vi "Actor Core.vi"(8 "error in":errorcluster caption="错误输入", 11 "Dialogue in":refnum<class "Dialogue.lvclass"> caption="操作者输入") -> (0 "error out":errorcluster caption="错误输出", 3 "Actor out":refnum<class "Actor.lvclass"> caption="操作者输出")   [LabVIEW 2014, in "Dialogue.lvlib" / "Dialogue.lvclass"]
doc: "(<B>文件名</B>：Actor Framework.lvlib:Actor.lvclass:Actor Core.vi)\n\n接收发送至操作者的消息，响应消息并处理可能导致操作者关闭的错误。\n\n子孙类重写该VI，使操作者完成特定的任务。使用调用父方法节点实现重写。"
uses:
  Dialogue.lvclass
  <vilib>/ActorFramework/Actor/Actor.lvclass
  <vilib>/ActorFramework/Actor/Actor.lvclass/Actor.ctl
  Dialogue.lvclass/Dialogue.ctl
  <vilib>/ActorFramework/Message Enqueuer/Message Enqueuer.lvclass/Message Enqueuer.ctl
  <vilib>/ActorFramework/Message Enqueuer/Enqueue.vi
  <vilib>/ActorFramework/Message Priority Queue/Priority Enqueue.vi
panel:
  out "格式化机器人指令":string[][](array[string])
  out "系统回应 4":string caption="标准输出"
  out "CM #":i32=-1
  out "显示窗口":string
  out "系统回应 3":string caption="标准输出"
  out "系统回应 2":string caption="标准输出"
  out "系统回应":string caption="标准输出"
  in  "重来":bool
  out "InstructionIn":string
  out "语音信号输出字符串":string
  in  "停止信号":bool
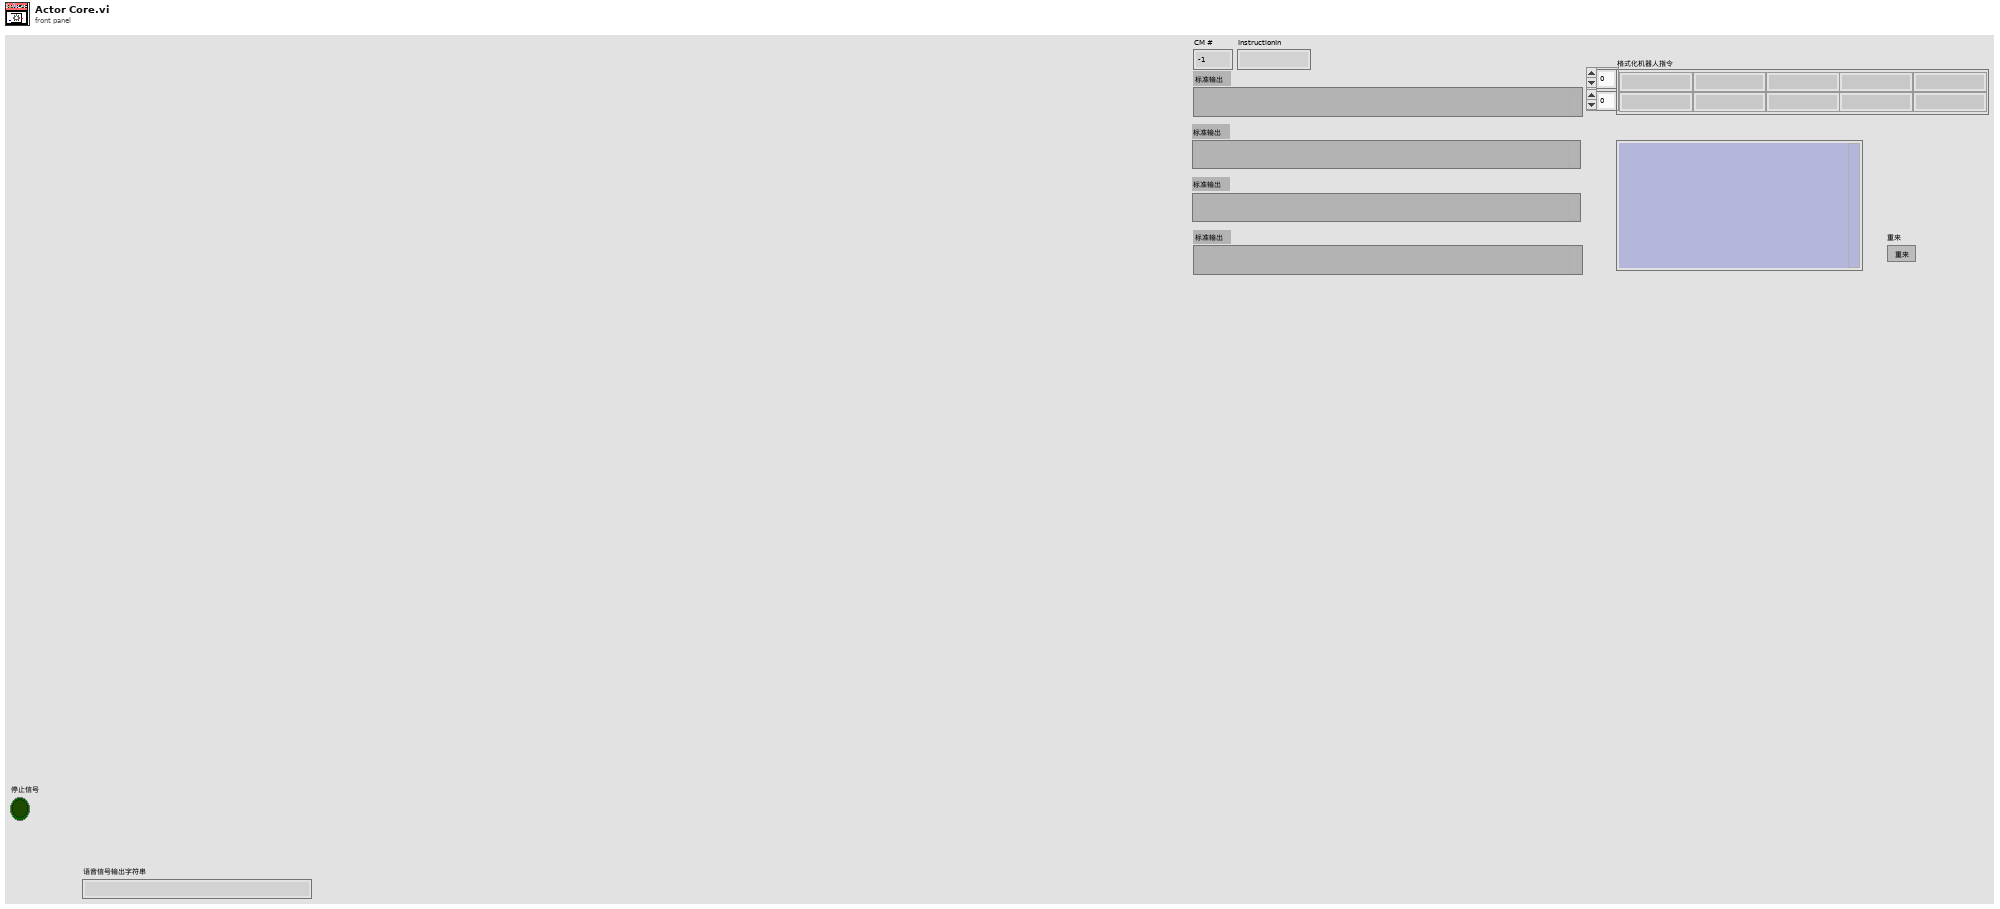
[diagram p1: front panel]
types:
  T1 = cluster{"输出数组":string[][], "CM #":i32, i32, string}
  T2 = cluster{"Stop":refnum<user-event>, "Text":refnum<user-event>, "Connected":refnum<user-event>}
  T3 = enum16{"open", "replace", "create", "open or create", "replace or create", "replace or create with confirmation"}
  T4 = cluster{"输出数组":string[][], "CM #":i32, "CM #":i32, string}
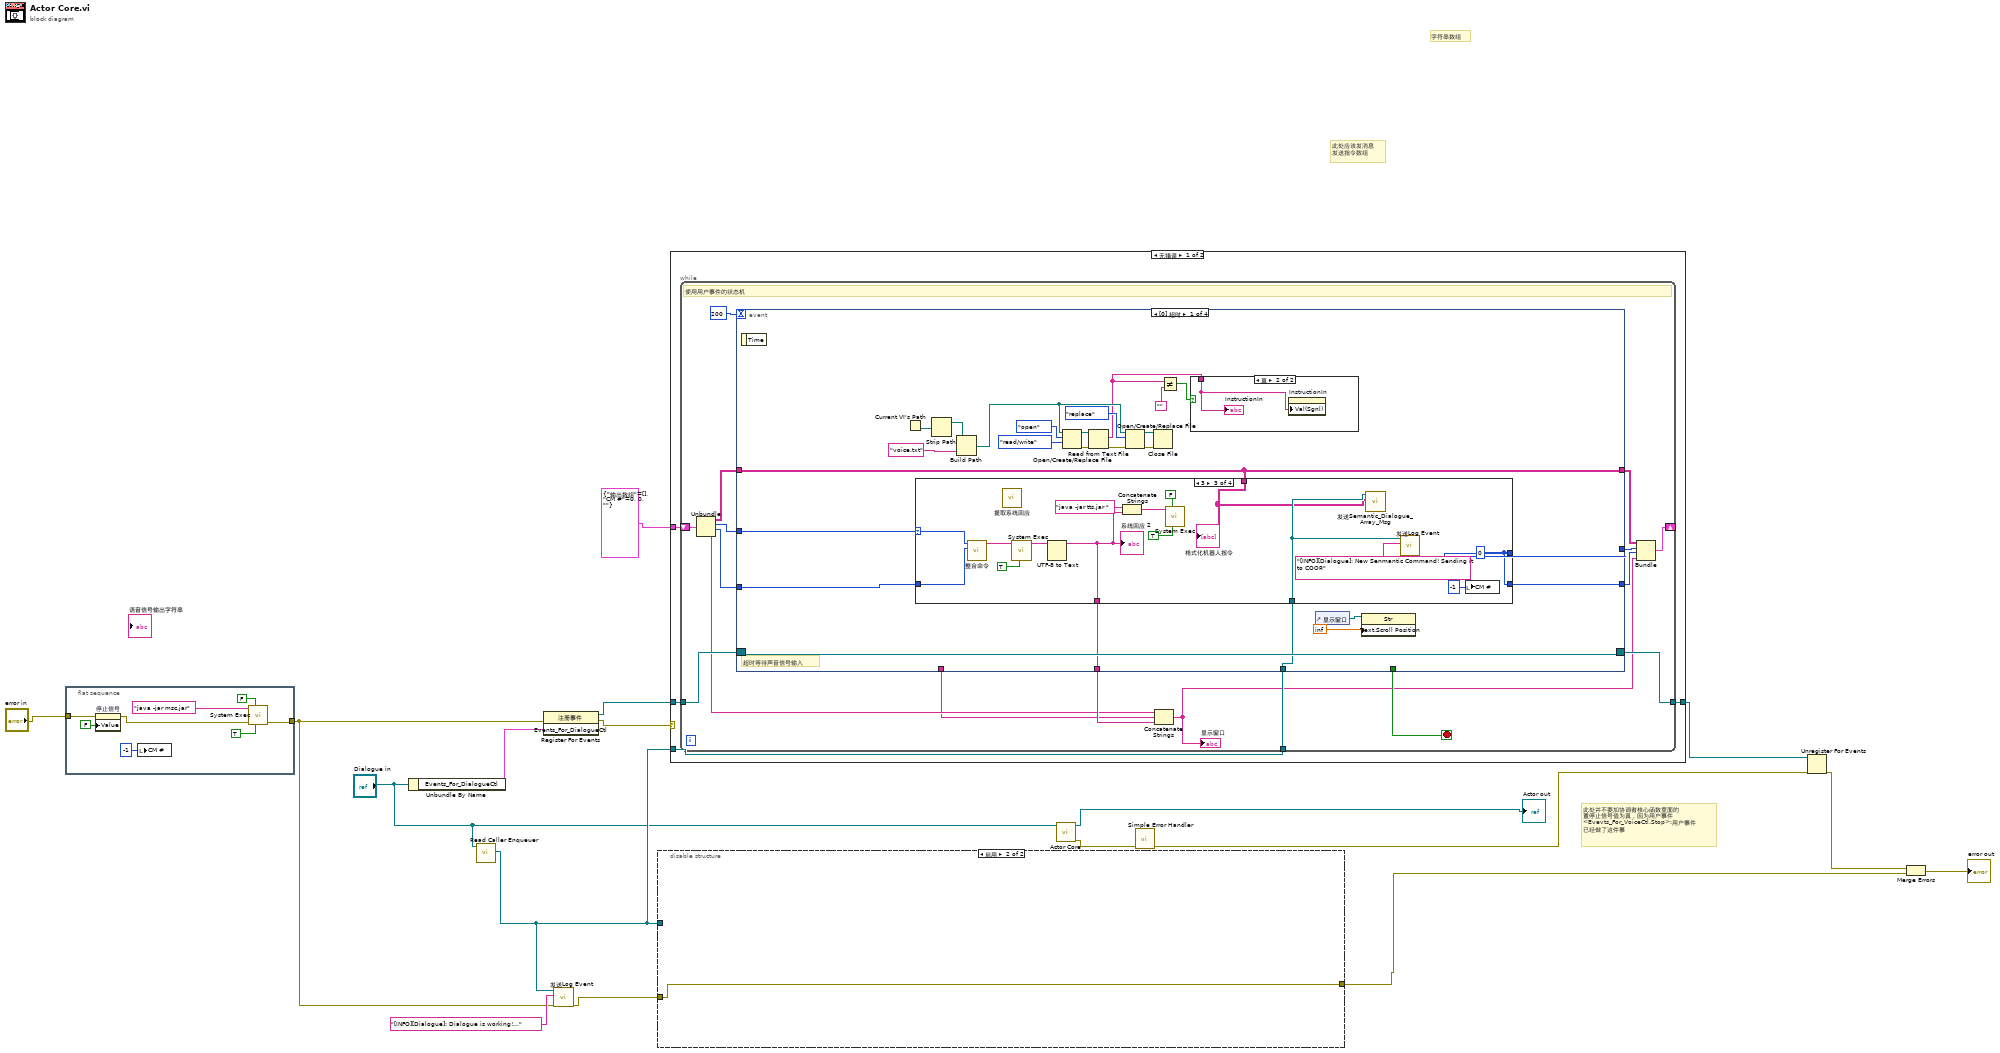
[diagram p0: block diagram]
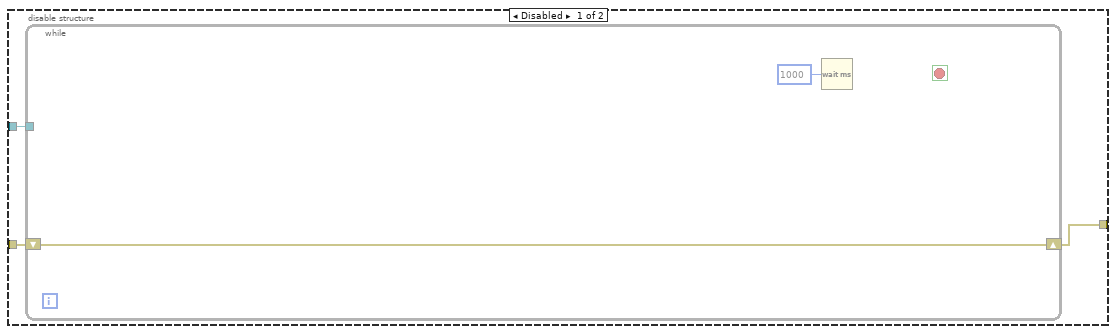
[diagram p2: hidden frame]
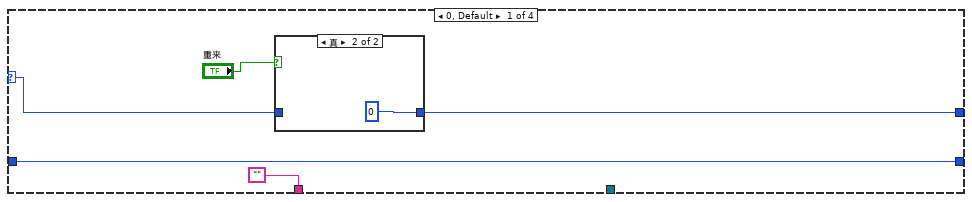
[diagram p3: hidden frame]
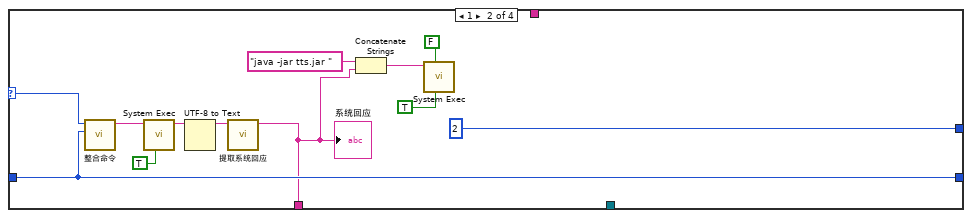
[diagram p5: hidden frame]
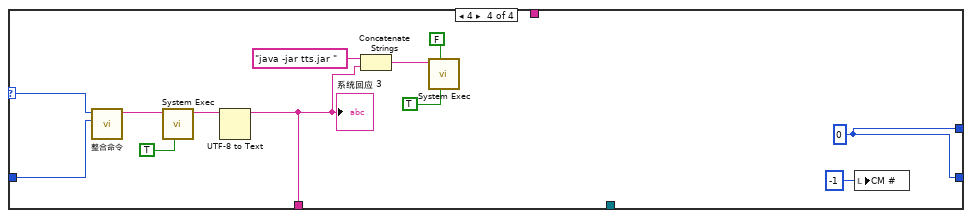
[diagram p6: hidden frame]
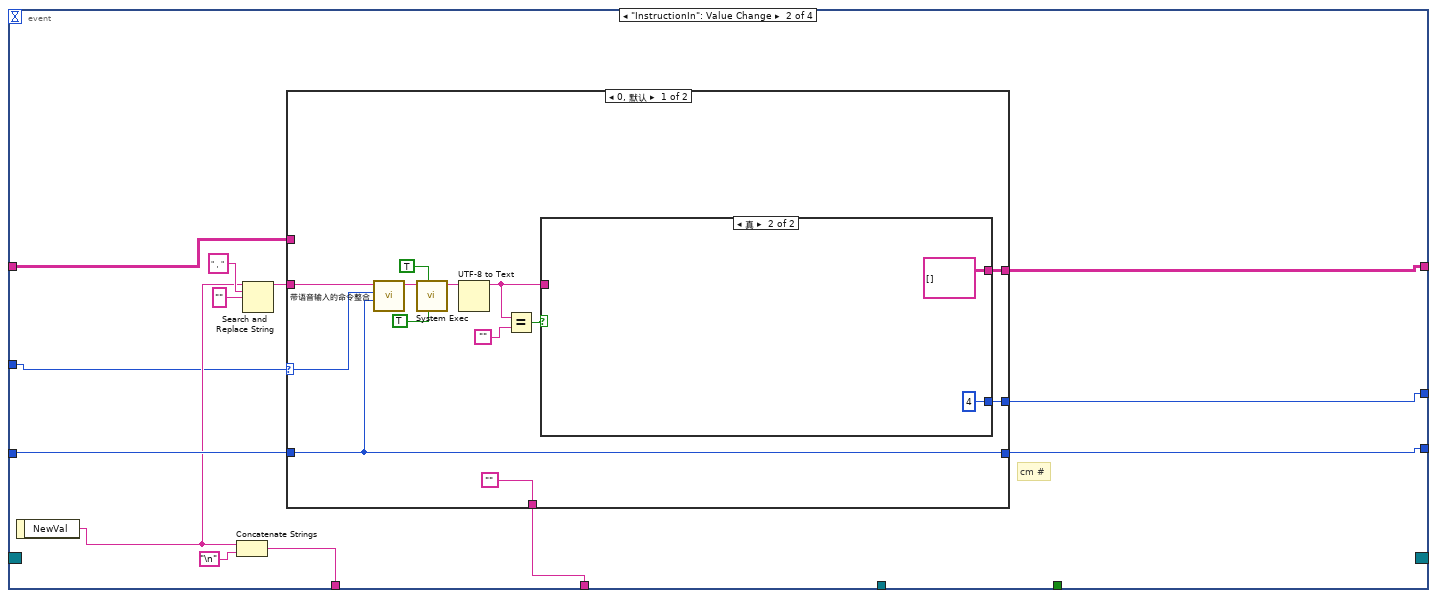
[diagram p8: hidden frame]
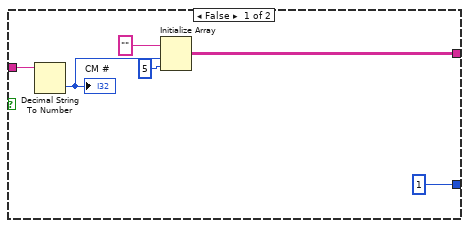
[diagram p9: hidden frame]
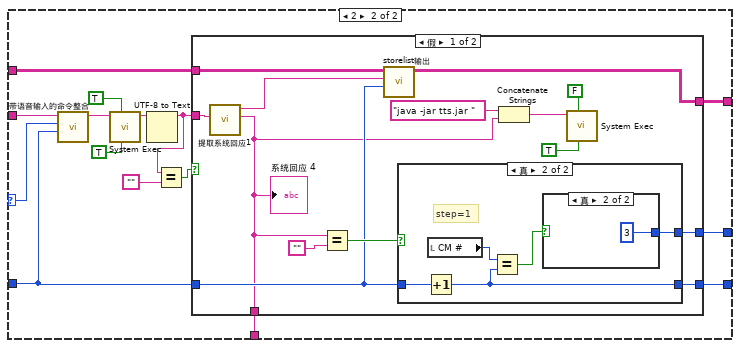
[diagram p10: hidden frame]
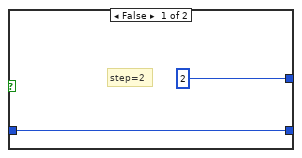
[diagram p11: hidden frame]
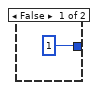
[diagram p12: hidden frame]
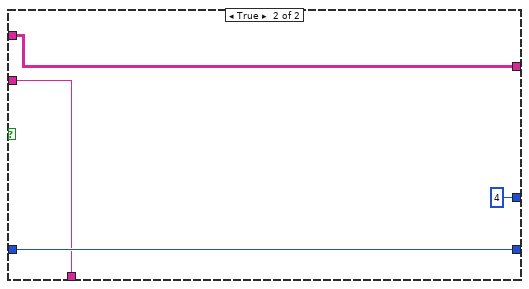
[diagram p13: hidden frame]
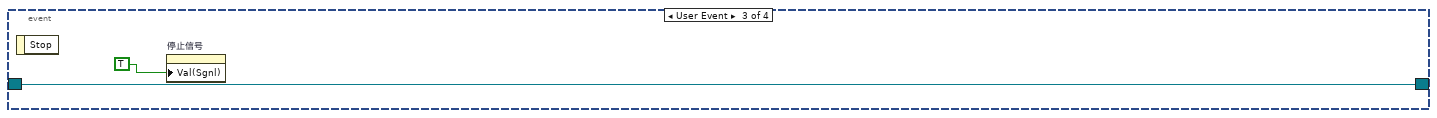
[diagram p14: hidden frame]
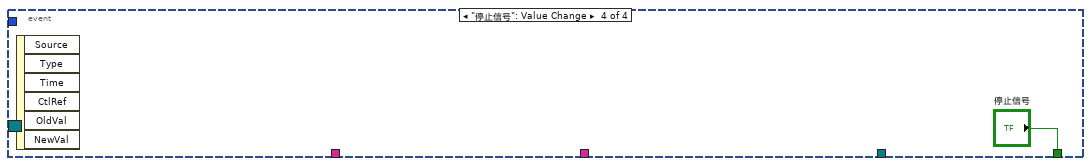
[diagram p15: hidden frame]
diagram:
  # "字符串数组"
  # "此处应该发消息\n发送指令数组"
  # "此处并不要加协调者核心函数里面的\n置停止信号值为真，因为用户事件\n<Evevts_For_VoiceCtl.Stop>:用户事件\n已经做了这件事"
  n1 = flat-sequence {
    tunnel: "error in" -> [w25]
    tunnel: [w19] -> w3
    frame #0 {
      n2 = property on="停止信号" class="Bool (严格)"(error in=w25, "Value"=FALSE ("停止信号")) -> (error out=w20:errorcluster)  [unwired: 1 in, 1 out]
      n3 = local write "CM #"(-1 ("CM #")) -> ()
      n4 = call <vilib>:"System Exec.vi"("run minimized? (F)"=TRUE, "wait until completion? (T)"=FALSE, "error in (no error)"=w20, "command line"="java -jar msc.jar") -> ("error out"=w19:errorcluster)  [unwired: 4 in, 3 out]
    }
  }
  n5 = Unbundle By Name("Dialogue in") -> ("Events_For_DialogueCtl"=w17:T2)
  n6 = call <vilib>:"Read Caller Enqueuer.vi"("Actor"="Dialogue in") -> ("Caller Enqueuer"=w9:refnum<class "Message Enqueuer.lvclass">)  [unwired: 10 in]
  n7 = register-events(error in=w3, w17) -> (reference out=w16:refnum<event-registration>, error out=w15:errorcluster)  [unwired: 1 in]
  n8 = call "发送Log Event.vi"("error in (no error)"=w3, "Event Text"="[INFO][Dialogue]: Dialogue is working!...", "消息待入队列"=w9) -> ("error out"=w10:cluster{"状态":bool, "代码":i32, "源":string})  [unwired: 7 in, 1 out]
  n9 = disable-structure shown="启用" {
    disable-tunnel: w10 -> [w28 w31]
    disable-tunnel: w9 -> [w27 _]
    disable-tunnel: [w26 w31] -> w2
    frame Disabled {
      n10 = while {
        tunnel: w27 -> [_]
        shift-right: [w29] -> w26
        shift-left: w28 -> [w29]
        stop <- _ stop-if-true
        n11 = Wait (ms)(milliseconds to wait=u32 1000 ("等待时间（毫秒）")) -> ()  [unwired: 1 out]
      }
    }
    frame Enabled {
    }
  }
  n12 = case shown="无错误" w15 {
    tunnel: [w35 w204] -> w12
    tunnel: w16 -> [w34 w204]
    tunnel: w9 -> [w33 _]
    tunnel: T1 {"输出数组"=[], "CM #"=0, 0, ""} -> [w32 _]
    frame No Error {
      n13 = while {
        tunnel: [w51] -> w35
        tunnel: w34 -> [w50]
        tunnel: w33 -> [w49]
        shift-right: [w39] -> _
        shift-left: w32 -> [w47]
        stop <- w52 stop-if-true
        # "使用用户事件的状态机"
        n14 = Unbundle(w47) -> ("输出数组"=w40:string[][], "CM #"=w41:i32, w42:i32, w37:string)
        n15 = event shown="[0] 超时" {
          selector: w50 -> [w77 _ w202 _]
          dyn-events: [w77 _ w202 _] -> w51
          timeout: 200 -> [_ _ _ _]
          tunnel: [_ _ _ "停止信号"] -> w52
          tunnel: w49 -> [w55 _ _ _]
          tunnel: w40 -> [w56 w128 _ _]
          tunnel: w41 -> [w61 w126 _ _]
          tunnel: w42 -> [w60 w130 _ _]
          tunnel: [w59 w125 _ _] -> w43
          tunnel: [w56 w133 _ _] -> w46
          tunnel: [w58 w132 _ _] -> w45
          tunnel: [w57 w131 _ _] -> w44
          tunnel: [_ w127 _ _] -> w36
          event Timeout {
            # "超时等待声音信号输入"
            n16 = event-data() -> ()  [unwired: 1 in, 1 out]
            n17 = Current VI's Path() -> (path=w76:path)
            n18 = case shown="3" w61 {
              selector: w61 -> [w78 w92 w109 w121]
              tunnel: [w79 2 w100 w113] -> w58
              tunnel: w60 -> [w81 w90 w107 w119]
              tunnel: ["" w85 w102 w114] -> w59
              tunnel: [w81 w90 w100 w113] -> w57
              tunnel: w56 -> [_ _ w97 _]
              tunnel: w55 -> [_ _ w98 _]
              frame 0, Default {
                n19 = case shown="真" "重来" {
                  tunnel: [w83 0] -> w79
                  tunnel: w78 -> [w83 _]
                  frame False {
                  }
                  frame True {
                  }
                }
              }
              frame 1 {
                n20 = call "整合命令.vi"("CM"=w90, "step"=w92) -> ("命令"=w91:string)  [unwired: 9 in]
                n21 = call <vilib>:"System Exec.vi"("run minimized? (F)"=TRUE, "command line"=w91) -> ("standard output"=w95:string)  [unwired: 6 in, 3 out]
                n22 = UTF-8 to Text(11:w95) -> (3:w94:string)  [unwired: 2 in, 1 out]
                n23 = call "提取系统回应.vi"("字符串"=w94) -> ("系统回应"=w85:string)  [unwired: 10 in]
                "系统回应" <- w85
                n24 = Concatenate Strings("java -jar tts.jar " ("command line"), w85) -> (w89:string)
                n25 = call <vilib>:"System Exec.vi"("run minimized? (F)"=TRUE, "wait until completion? (T)"=FALSE, "command line"=w89) -> ()  [unwired: 5 in, 4 out]
              }
              frame 3 {
                w100 = 0 ("CM #")
                n26 = call "整合命令.vi"("CM"=w107, "step"=w109) -> ("命令"=w108:string)  [unwired: 9 in]
                n27 = call "提取系统回应.vi"() -> ()  [unwired: 11 in, 1 out]
                n28 = call <vilib>:"System Exec.vi"("run minimized? (F)"=TRUE, "command line"=w108) -> ("standard output"=w111:string)  [unwired: 6 in, 3 out]
                n29 = UTF-8 to Text(11:w111) -> (3:w102:string)  [unwired: 2 in, 1 out]
                "系统回应 2" <- w102
                n30 = Concatenate Strings("java -jar tts.jar " ("command line"), w102) -> (w106:string)
                n31 = call <vilib>:"System Exec.vi"("run minimized? (F)"=TRUE, "wait until completion? (T)"=FALSE, "command line"=w106) -> ()  [unwired: 5 in, 4 out]
                n32 = call "发送Semantic_Dialogue_Array_Msg.vi"("值(信号)"=w97, "消息待入队列"=w98) -> ()  [unwired: 8 in, 2 out]
                n33 = call "发送Log Event.vi"("Event Text"="[INFO][Dialogue]: New Senmantic Command! Sending it to COOR", "消息待入队列"=w98) -> ()  [unwired: 8 in, 2 out]
                n34 = local write "CM #"(-1 ("CM #")) -> ()
                "格式化机器人指令" <- w97
              }
              frame 4 {
                w113 = 0 ("CM #")
                n35 = call "整合命令.vi"("CM"=w119, "step"=w121) -> ("命令"=w120:string)  [unwired: 9 in]
                n36 = call <vilib>:"System Exec.vi"("run minimized? (F)"=TRUE, "command line"=w120) -> ("standard output"=w123:string)  [unwired: 6 in, 3 out]
                n37 = UTF-8 to Text(11:w123) -> (3:w114:string)  [unwired: 2 in, 1 out]
                "系统回应 3" <- w114
                n38 = Concatenate Strings("java -jar tts.jar " ("command line"), w114) -> (w118:string)
                n39 = call <vilib>:"System Exec.vi"("run minimized? (F)"=TRUE, "wait until completion? (T)"=FALSE, "command line"=w118) -> ()  [unwired: 5 in, 4 out]
                n40 = local write "CM #"(-1 ("CM #")) -> ()
              }
            }
            n41 = Strip Path(path=w76) -> (stripped path=w73:path)  [unwired: 1 out]
            n42 = Build Path(base path=w73, name or relative path="voice.txt" ("名称或相对路径")) -> (appended path=w75:path)
            n43 = Open/Create/Replace File(file path (use dialog)=w75, operation (0:open)=T3."open" ("操作(0:open)"), access (0:read/write)=enum16{"read/write", "read-only", "write-only"}."read/write" ("权限(0:read/write)")) -> (refnum out=w68:refnum<file>, error out=w67:errorcluster)  [unwired: 3 in, 1 out]
            n44 = Read from Text File(file (use dialog)=w68, error in=w67) -> (text=w62:string, error out=w70:errorcluster)  [unwired: 2 in, 2 out]
            n45 = Open/Create/Replace File(file path (use dialog)=w75, error in=w70, operation (0:open)=T3."replace" ("操作(0:open)")) -> (refnum out=w71:refnum<file>, error out=w72:errorcluster)  [unwired: 3 in, 1 out]
            n46 = Close File(refnum=w71, error in=w72) -> ()  [unwired: 2 out]
            n47 = Not Equal?(x=w62, y="") -> (x != y?=w63:bool)
            n48 = case shown="真" w63 {
              tunnel: w62 -> [_ w124]
              frame False {
              }
              frame True {
                n49 = property on="InstructionIn" class="Str"("Val(Sgnl)"=w124) -> ()  [unwired: 2 in, 2 out]
                "InstructionIn" <- w124
              }
            }
            n50 = control-ref of="显示窗口"() -> (w54:refnum<vi>)
            n51 = property on="属性节点" class="Str"(reference=w54, "Text.Scroll Position"=inf) -> ()  [unwired: 1 in, 2 out]
          }
          event "InstructionIn": Value Change {
            # "cm #"
            n52 = event-data() -> ("NewVal"=w129:string)  [unwired: 1 in]
            n53 = Concatenate Strings(w129, "\n") -> (w127:string)
            n54 = Search and Replace String(input string=w129, search string="，" ("子字符串(\"\")"), replace string="" ("替换字符串(\"\")")) -> (result string=w134:string)  [unwired: 5 in, 3 out]
            n55 = case shown="0, 默认" w126 {
              selector: w126 -> [w145 w167]
              tunnel: [w144 w171] -> w131
              tunnel: w130 -> [w144 w164]
              tunnel: [w148 w170] -> w132
              tunnel: ["" w165] -> w125
              tunnel: w134 -> [w143 w168]
              tunnel: [w141 w162] -> w133
              tunnel: w128 -> [_ w163]
              frame 0, Default {
                n56 = call "带语音输入的命令整合.vi"("CM"=w144, "step"=w145, "输入指令"=w143) -> ("命令"=w142:string)  [unwired: 8 in]
                n57 = call <vilib>:"System Exec.vi"("run minimized? (F)"=TRUE, "wait until completion? (T)"=TRUE, "command line"=w142) -> ("standard output"=w149:string)  [unwired: 5 in, 3 out]
                n58 = UTF-8 to Text(11:w149) -> (3:w139:string)  [unwired: 2 in, 1 out]
                n59 = Equal?(x=w139, y="") -> (x = y?=w138:bool)
                n60 = case shown="真" w138 {
                  tunnel: [1 4] -> w148
                  tunnel: w139 -> [w155 _]
                  tunnel: [w151 string[][] []] -> w141
                  frame False {
                    n61 = Decimal String To Number(string=w155) -> (number=w153:i32)  [unwired: 2 in, 1 out]
                    "CM #" <- w153
                    n62 = Initialize Array("", w153, 5 ("维数大小")) -> (w151:string[][])
                  }
                  frame True {
                  }
                }
              }
              frame 2 {
                n63 = call "带语音输入的命令整合.vi"("CM"=w164, "step"=w167, "输入指令"=w168) -> ("命令"=w166:string)  [unwired: 8 in]
                n64 = call <vilib>:"System Exec.vi"("run minimized? (F)"=TRUE, "wait until completion? (T)"=TRUE, "command line"=w166) -> ("standard output"=w172:string)  [unwired: 5 in, 3 out]
                n65 = UTF-8 to Text(11:w172) -> (3:w160:string)  [unwired: 2 in, 1 out]
                n66 = Equal?(x=w160, y="") -> (x = y?=w159:bool)
                n67 = case shown="假" w159 {
                  tunnel: [w185 w200] -> w171
                  tunnel: [w184 4] -> w170
                  tunnel: w160 -> [w183 w197]
                  tunnel: [w174 w197] -> w165
                  tunnel: w164 -> [w181 w200]
                  tunnel: w163 -> [w180 w198]
                  tunnel: [w179 w198] -> w162
                  frame False {
                    n68 = call "提取系统回应1.vi"("字符串"=w183) -> ("系统回应"=w174:string, "子字符串之前"=w182:string)  [unwired: 9 in]
                    "系统回应 4" <- w174
                    n69 = Equal?(x=w174, y="") -> (x = y?=w186:bool)
                    n70 = call "storelist输出.vi"("CM"=w181, 10:"storelist"=w182, 11:"storelist"=w180) -> ("输出数组"=w179:string[][])  [unwired: 8 in]
                    n71 = case shown="真" w186 {
                      tunnel: [2 w193] -> w184
                      tunnel: w181 -> [w189 w194]
                      tunnel: [w189 w190] -> w185
                      frame False {
                        # "step=2"
                      }
                      frame True {
                        # "step=1"
                        n72 = Increment(x=w194) -> (x+1=w190:i32)
                        n73 = local read "CM #"() -> (w192:i32)
                        n74 = Equal?(x=w192, y=w190) -> (x = y?=w191:bool)
                        n75 = case shown="真" w191 {
                          tunnel: [1 3] -> w193
                          frame False {
                          }
                          frame True {
                          }
                        }
                      }
                    }
                    n76 = Concatenate Strings("java -jar tts.jar " ("command line"), w174) -> (w178:string)
                    n77 = call <vilib>:"System Exec.vi"("run minimized? (F)"=TRUE, "wait until completion? (T)"=FALSE, "command line"=w178) -> ()  [unwired: 5 in, 4 out]
                  }
                  frame True {
                  }
                }
              }
            }
          }
          event User Event {
            n78 = event-data() -> ()  [unwired: 1 in, 1 out]
            n79 = property on="停止信号" class="Bool (严格)"("Val(Sgnl)"=TRUE) -> ()  [unwired: 2 in, 2 out]
          }
          event "停止信号": Value Change {
            n80 = event-data() -> ()  [unwired: 1 in, 6 out]
          }
        }
        n81 = Concatenate Strings(w37, w36, w43) -> (w38:string)
        "显示窗口" <- w38
        n82 = Bundle("输出数组"=w46, "CM #"=w45, "CM #"=w44, w38) -> (w39:T4)  [unwired: 1 in]
      }
    }
    frame Error {
    }
  }
  n83 = call-parent "Actor Core.vi"("Actor in"="Dialogue in") -> ("error out"=w14:errorcluster, "Actor out"=→"Actor out":refnum<class "Actor.lvclass">)  [unwired: 9 in]
  n84 = call <vilib>:"Simple Error Handler.vi"("error in (no error)"=w14) -> ("error out"=w13:errorcluster)  [unwired: 4 in, 4 out]
  n85 = Unregister For Events(event registration refnum=w12, error in=w13) -> (error out=w11:errorcluster)
  n86 = Merge Errors(w11, w2) -> (→"error out":errorcluster)
